vi "__vna_set_constant_frequency_mode.vi"(3 "error in (no error)":errorcluster, 4 "Power dBm":dbl=-25.0 caption="Power, dBm" format="%#.3f", 5 "Center Freq (Hz):":dbl=3090000000.0 format="%#.6f") -> (0 "error out":errorcluster)   [LabVIEW 2013]
uses:
  <instrlib>/Rohde&Schwarz Vector Network Analyzer/Rohde&Schwarz Vector Network Analyzer.lvlib
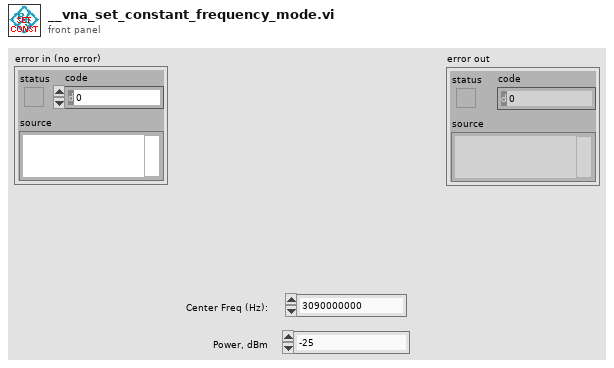
[diagram p1: front panel]
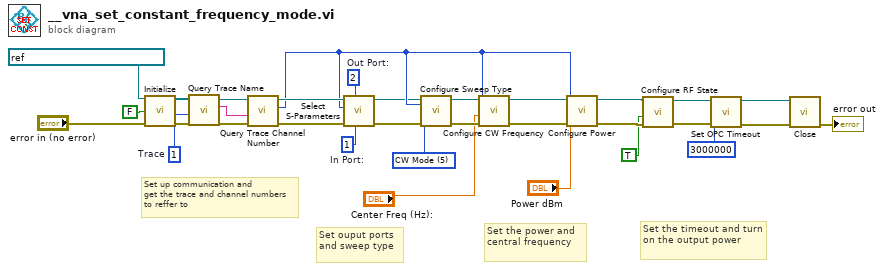
[diagram p0: block diagram]
diagram:
  w14 = 5 items=["Lin. Frequency", "Log. Frequency", "Segmented Frequency", "Power", "Time", "CW Mode"] ("Sweep Type (Power)")
  w22 = 1  # Trace
  w21 = 1  # In Port:
  w20 = 2  # Out Port:
  # "Set the timeout and turn on the output power"
  # "Set the power and central frequency"
  # "Set ouput ports and sweep type"
  # "Set up communication and\nget the trace and channel numbers\nto reffer to"
  n1 = call <instrlib>:"Initialize.vi"("VISA resource name"=refnum<visa-resource-name> "TCPIP::192.168.0.3::INST", "Reset (T: Reset)"=FALSE, "error in (no error)"="error in (no error)") -> ("VISA resource name out"=w27:refnum<visa-resource-name>, "error out"=w28:errorcluster)  [unwired: 11 in]
  n2 = call <instrlib>:"Query Trace Name.vi"("error in (no error)"=w28, "Trace Number (1)"=w22, "VISA resource name"=w27) -> ("error out"=w30:errorcluster, "Trace Name"=w19:string, "VISA resource name out"=w29:refnum<visa-resource-name>)  [unwired: 6 in]
  n3 = call <instrlib>:"Query Trace Channel Number.vi"("error in (no error)"=w30, "Trace Name (\"Ch2Trc2\")"=w19, "VISA resource name"=w29) -> ("error out"=w32:errorcluster, "Channel Number"=w18:i32, "VISA resource name out"=w31:refnum<visa-resource-name>)  [unwired: 6 in]
  n4 = call <instrlib>:"Select S-Parameters.vi"("In Port (1)"=w21, "Out Port (1)"=w20, "error in (no error)"=w32, "Channel (1)"=w18, "VISA resource name"=w31) -> ("error out"=w12:errorcluster, "VISA resource name out"=w13:refnum<visa-resource-name>)  [unwired: 5 in]
  n5 = call <instrlib>:"Configure Sweep Type.vi"("error in (no error)"=w12, "Sweep Type (Power)"=w14, "Channel (1)"=w18, "VISA resource name"=w13) -> ("error out"=w16:errorcluster, "VISA resource name out"=w17:refnum<visa-resource-name>)  [unwired: 6 in]
  n6 = call <instrlib>:"Configure CW Frequency.vi"("error in (no error)"=w16, "CW Frequency (1.0e9)"="Center Freq (Hz):", "Channel (1)"=w18, "VISA resource name"=w17) -> ("error out"=w24:errorcluster, "VISA resource name out"=w25:refnum<visa-resource-name>)  [unwired: 6 in]
  n7 = call <instrlib>:"Configure Power.vi"("error in (no error)"=w24, "Power (-10.0)"="Power dBm", "Channel (1)"=w18, "VISA resource name"=w25) -> ("error out"=w10:errorcluster, "VISA resource name out"=w7:refnum<visa-resource-name>)  [unwired: 6 in]
  n8 = call <instrlib>:"Configure RF State.vi"("error in (no error)"=w10, "RF State (T)"=TRUE, "VISA resource name"=w7) -> ("error out"=w9:errorcluster, "VISA resource name out"=w8:refnum<visa-resource-name>)  [unwired: 7 in]
  n9 = call <instrlib>:"Set OPC Timeout.vi"("error in (no error)"=w9, "OPC Timeout (30000)"=3000000, "VISA resource name"=w8) -> ("error out"=w4:errorcluster, "VISA resource name out"=w5:refnum<visa-resource-name>)  [unwired: 7 in]
  n10 = call <instrlib>:"Close.vi"("error in (no error)"=w4, "VISA resource name"=w5) -> ("error out"=→"error out":errorcluster)  [unwired: 9 in]
